vi "SVI_ExtractReadings.vi"(11 "read buffer":string) -> (2 "Current":dbl, 3 "Scan Voltage (V)":dbl)   [LabVIEW 2014]
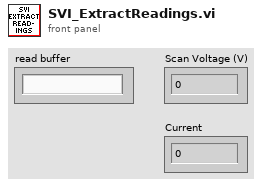
[diagram p1: front panel]
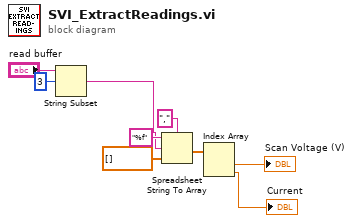
[diagram p0: block diagram]
diagram:
  n1 = String Subset(string="read buffer", offset (0)=3) -> (substring=w7:string)  [unwired: 1 in]
  n2 = Spreadsheet String To Array(delimiter (Tab)=",", format string="%f", spreadsheet string=w7, array type (2D Dbl)=dbl[] []) -> (array=w4:dbl[])
  n3 = Index Array(array=w4) -> (element #1=→"Scan Voltage (V)":dbl, element #2=→"Current":dbl)  [unwired: 2 in]
